vi "Error To Log.vi"(11 "error in (no error)":errorcluster) -> (15 "error out":errorcluster)   [LabVIEW 2018]
uses:
  Logger/Log File Input.ctl
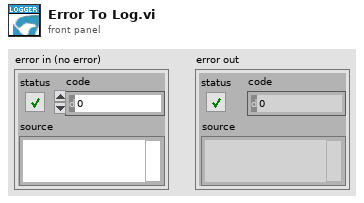
[diagram p1: front panel]
types:
  T1 = typedef "Log File Input.ctl" = cluster{"Log File Input":string, "Log Entry Type":enum16{"STANDARD", "WARNING", "CRITICAL"}}
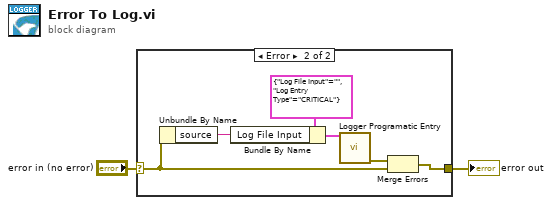
[diagram p0: block diagram]
diagram:
  n1 = case shown="Error" "error in (no error)" {
    selector: "error in (no error)" -> [w3 w5]
    tunnel: [w3 w9] -> w1
    frame No Error {
    }
    frame Error {
      n2 = Unbundle By Name(w5) -> ("source"=w4:string)
      n3 = Bundle By Name(cluster=T1 {"Log File Input"="", "Log Entry Type"=enum."CRITICAL"} ("Log File Input"), "Log File Input"=w4) -> (w7:T1)
      n4 = call "Logger Programatic Entry.vi"("Log File Input"=w7) -> ("error out"=w8:errorcluster)  [unwired: 14 in]
      n5 = Merge Errors(w8, w5) -> (w9:errorcluster)
    }
  }
  "error out" <- w1
